vi "WriteSystemData.vi"(8 "error in (no error)":errorcluster, 10 "SystemDataCluster":T1 {"FFTmagnitudes"."magnitude" format="%.2p"; "FFTmagnitudes"."f0" format="%.2p"; "FFTmagnitudes"."df" format="%.2p"}, 11 "Data Value Reference IN":refnum<data-value>) -> (0 "error out":errorcluster, 3 "Data Value Reference out":refnum<data-value>)   [LabVIEW 2013]
uses:
  Control/SystemData.ctl
  Control/SignalType.ctl
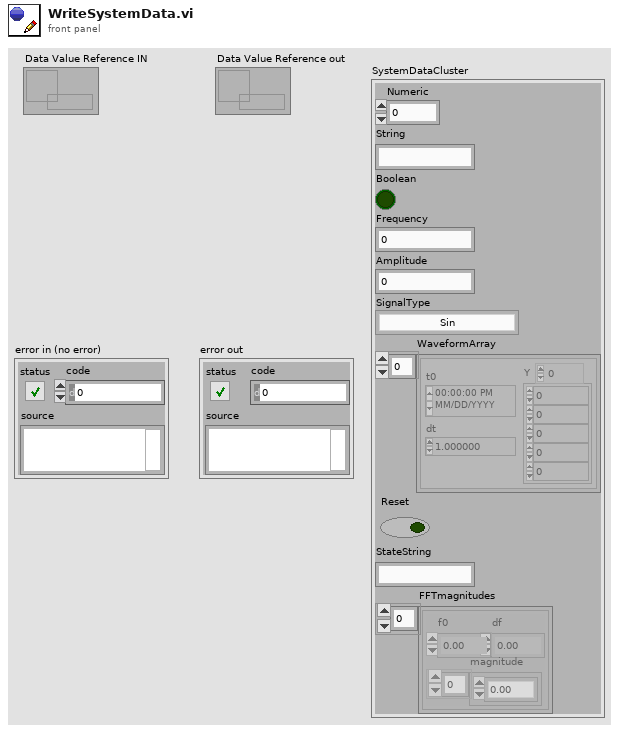
[diagram p1: front panel]
types:
  T1 = typedef "SystemData.ctl" = cluster{"Numeric":dbl, "String":string, "Boolean":bool, "Frequency":dbl, "Amplitude":dbl, "SignalType":T2, "WaveformArray":waveform(dbl)[], "Reset":bool, "StateString":string, "FFTmagnitudes":cluster{"f0":dbl, "df":dbl, "magnitude":dbl[]}[]}
  T2 = typedef "SignalType.ctl" = enum16{"Sin", "Triangle", "Square"}
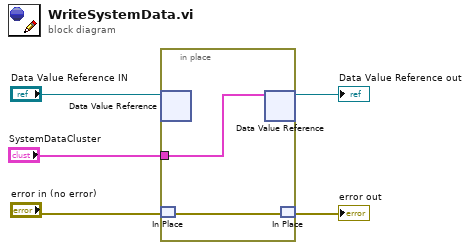
[diagram p0: block diagram]
diagram:
  n1 = in-place {
    in-place-border: "SystemDataCluster" -> [w6]
    n2 = in-place-dvr #1("Data Value Reference IN") -> ()  [unwired: 2 out]
    n3 = in-place-match #2("error in (no error)") -> (w7:errorcluster)
    n4 = in-place-dvr #1(w6) -> (→"Data Value Reference out":refnum<data-value>)  [unwired: 1 out]
    n5 = in-place-match #2(w7) -> (→"error out":errorcluster)
  }
